vi "Generate Iota RC Array.vi"() -> (0 "iota rc array":T1[](array[typedef]) format="%016x")   [LabVIEW 2020, in "NI_Keccak.lvlib"]
uses:
  <vilib>/security/Message Digest/Keccak/NI_Keccak.lvlib
  <vilib>/security/Message Digest/SHA-3/subVIs/state word.ctl
  <vilib>/security/Message Digest/SHA-3/NI_SHA-3.lvclass
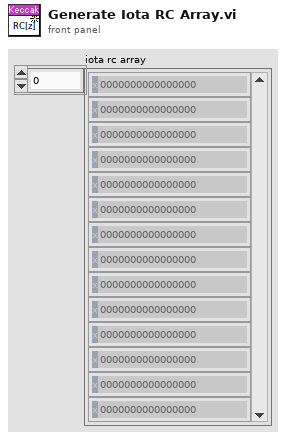
[diagram p1: front panel]
types:
  T1 = typedef "NI_SHA-3.lvclass/state word.ctl" = u64
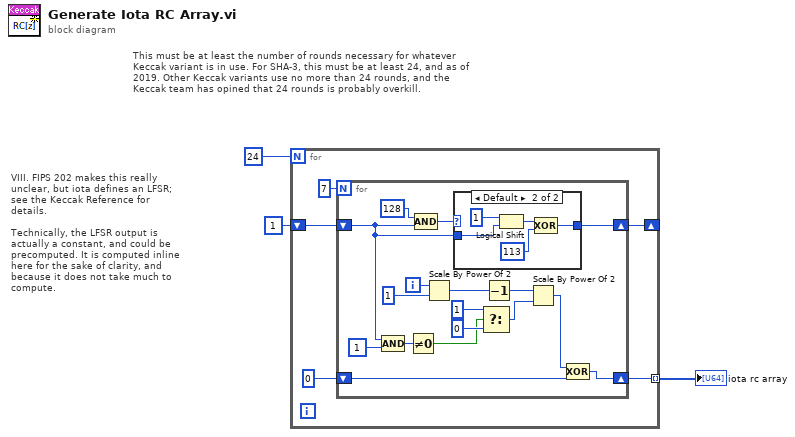
[diagram p0: block diagram]
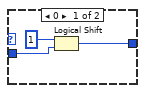
[diagram p2: hidden frame]
diagram:
  # "VIII. FIPS 202 makes this really unclear, but iota defines an LFSR; see the Keccak Reference for details.\n\nTechnically, the LFSR output is actually a constant, and could be precomputed. It is computed inline here for the sake of clarity, and because it does not take much to compute."
  # "This must be at least the number of rounds necessary for whatever Keccak variant is in use. For SHA-3, this must be at least 24, and as of 2019. Other Keccak variants use no more than 24 rounds, and the Keccak team has opined that 24 rounds is probably overkill."
  n1 = for {
    N: 24 -> [_]
    tunnel: [w4] -> w3 mode=indexing
    shift-right: [w6] -> _
    shift-left: u8 1 ("lfsr in") -> [w7]
    n2 = for {
      N: 7 -> [_]
      shift-right: [w15] -> w6
      shift-left: w7 -> [w14]
      shift-right: [w10] -> w4
      shift-left: T1 0 ("value") -> [w9]
      i -> [w25]
      n3 = Compound Arithmetic op=AND(w14, u8 1 ("value")) -> (w19:u8)
      n4 = Not Equal To 0?(x=w19) -> (x != 0?=w18:bool)
      n5 = Compound Arithmetic op=AND(u8 128 ("value"), w14) -> (w16:u8)
      n6 = Scale By Power Of 2(n=w25, x=1) -> (x*2^n=w23:i32)
      n7 = case shown="Default" w16 {
        tunnel: w14 -> [w28 w33]
        tunnel: [w26 w29] -> w15
        frame 0 {
          n8 = Logical Shift(y=i16 1, x=w28) -> (x << y=w26:u8)
        }
        frame Default {
          n9 = Logical Shift(y=i16 1, x=w33) -> (x << y=w31:u8)
          n10 = Compound Arithmetic op=XOR(w31, u8 113 ("value")) -> (w29:u8)
        }
      }
      n11 = Select(t=T1 1, s=w18, f=T1 0) -> (s? t:f=w12:T1)
      n12 = Decrement(x=w23) -> (x-1=w13:i32)
      n13 = Scale By Power Of 2(n=w13, x=w12) -> (x*2^n=w11:T1)
      n14 = Compound Arithmetic op=XOR(w11, w9) -> (w10:T1)
    }
  }
  "iota rc array" <- w3
